vi "Tree Get Current.vi"(8 "error in (no error)":errorcluster, 10 "Tree name":string, 11 "Tree DVR in":refnum<data-value>) -> (0 "error out":errorcluster, 2 "Current shot out":i32, 3 "Tree DVR out":refnum<data-value>)   [LabVIEW 2010, in "MDSplus.lvlib"]
doc: "Return the current shot for that tree."
uses:
  <vilib>/MDSplus/Library/MDSplus.lvlib
  <vilib>/MDSplus/Classes/Tree_Class/Tree.lvclass
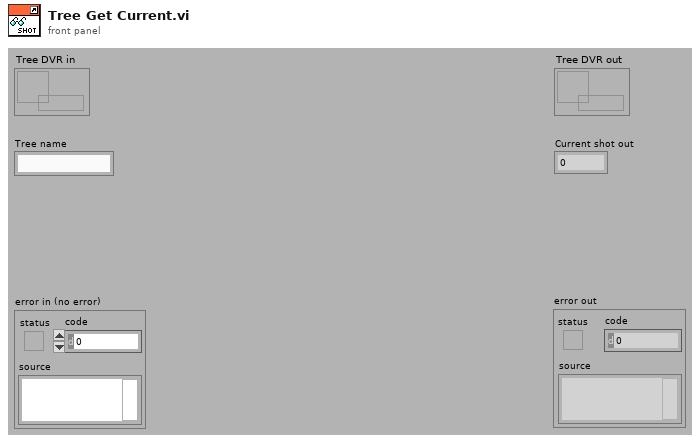
[diagram p1: front panel]
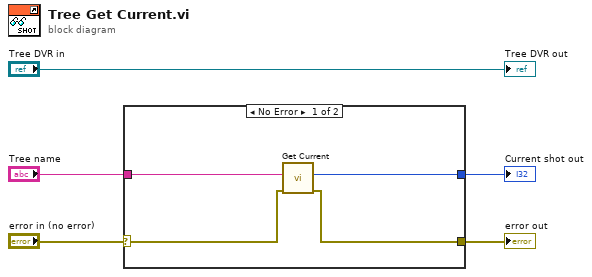
[diagram p0: block diagram]
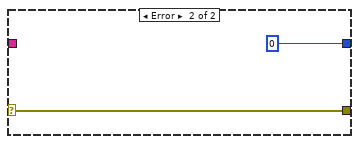
[diagram p2: hidden frame]
diagram:
  n1 = case shown="No Error" "error in (no error)" {
    selector: "error in (no error)" -> [w8 w11]
    tunnel: [w7 w11] -> w5
    tunnel: [w6 0 ("Size out")] -> w3
    tunnel: "Tree name" -> [w9 _]
    frame No Error {
      n2 = call <vilib>:"Get Current.vi"("error in (no error)"=w8, "Tree name"=w9) -> ("error out"=w7:errorcluster, "Current shot out"=w6:i32)  [unwired: 7 in, 1 out]
    }
    frame Error {
    }
  }
  "error out" <- w5
  "Current shot out" <- w3
  "Tree DVR out" <- "Tree DVR in"
